vi "ATReadErds.vi"(0 "GEA2 Reference In":refnum<k24>, 5 "Destination":string, 7 "Erd Number":string, 11 "Error In":errorcluster) -> (4 "GEA2 Reference Out":refnum<k24>, 8 "ERD Data Out":string, 15 "Error Out":errorcluster)   [LabVIEW 2021]
uses:
  D:/Common/LabVIEW GEA2 Toolkit/source/GEA3 DLL Source/GeaCommunication.dll
  Common/LabVIEW GEA2 Toolkit/source/GEA3 DLL Source/GeaCommunication.dll
  Common/LabVIEW GEA2 Toolkit/GEA3/type defs/Data Type.ctl
  Common/LabVIEW GEA2 Toolkit/GEA3/library/GEA2_Toolkit.lvlib
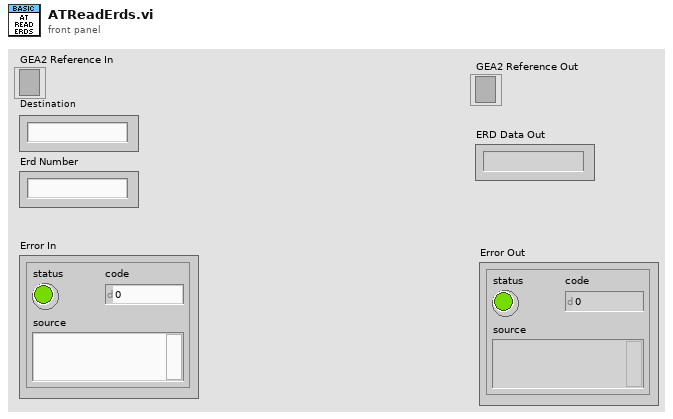
[diagram p1: front panel]
types:
  T1 = typedef "Data Type.ctl" = enum16{"string", "boolean", "uint8_t", "uint16_t", "uint32_t", "uint64_t", "int8_t", "int16_t", "int32_t", "int64_t"}
  T2 = cluster{"ERD Data Out[0]":cluster{"ERD Number":u16, "Data":string}, "ERD Data Out[1]":cluster{"ERD Number":u16, "Data":string}, "ERD Data Out[2]":cluster{"ERD Number":u16, "Data":string}, "ERD Data Out[3]":cluster{"ERD Number":u16, "Data":string}, "ERD Data Out[4]":cluster{"ERD Number":u16, "Data":string}, "ERD Data Out[5]":cluster{"ERD Number":u16, "Data":string}, "ERD Data Out[6]":cluster{"ERD Number":u16, "Data":string}, "ERD Data Out[7]":cluster{"ERD Number":u16, "Data":string}, "ERD Data Out[8]":cluster{"ERD Number":u16, "Data":string}}
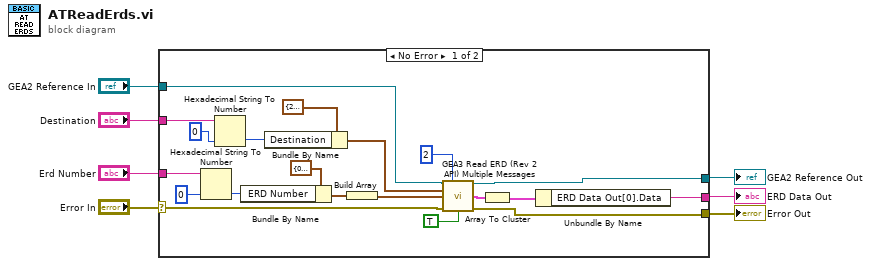
[diagram p0: block diagram]
diagram:
  n1 = case shown="No Error" "Error In" {
    selector: "Error In" -> [w12 w29]
    tunnel: "GEA2 Reference In" -> [w16 w28]
    tunnel: "Destination" -> [w20 _]
    tunnel: "Erd Number" -> [w19 _]
    tunnel: [w15 w28] -> w4
    tunnel: [w17 _] -> w3
    tunnel: [w13 w29] -> w1
    frame No Error {
      n2 = Hexadecimal String To Number(string=w19, default (0uL)=u16 0 ("ERD Number")) -> (number=w23:u16)  [unwired: 1 in, 1 out]
      n3 = Hexadecimal String To Number(string=w20, default (0uL)=u8 0 ("Destination")) -> (number=w26:u8)  [unwired: 1 in, 1 out]
      n4 = Bundle By Name(cluster=cluster{"ERD Number":u16, "Data Type":T1} {"ERD Number"=0, "Data Type"=enum."string"} ("ERD Read Data In"), "ERD Number"=w23) -> (w21:cluster{"ERD Number":u16, "Data Type":T1})
      n5 = Bundle By Name(cluster=cluster{"Source":u8, "Destination":u8} {"Source"=229, "Destination"=0} ("GEA Inputs"), "Destination"=w26) -> (w10:cluster{"Source":u8, "Destination":u8})
      n6 = Build Array(w21) -> (w11:cluster{"ERD Number":u16, "Data Type":T1}[])
      n7 = call "GEA3 Read ERD (Rev 2 API) Multiple Messages.vi"("GEA2 Reference In"=w16, "Retry Count"=2, "GEA Inputs"=w10, "Read ERD List"=w11, "Error In"=w12, "Verify ERD Response?"=TRUE) -> ("GEA2 Reference Out"=w15:refnum<k24>, "ERD Data Out"=w14:cluster{"ERD Number":u16, "Data":string}[], "Error Out"=w13:errorcluster)  [unwired: 6 in, 1 out]
      n8 = Array To Cluster(array=w14) -> (cluster=w18:T2)
      n9 = Unbundle By Name(w18) -> ("ERD Data Out[0].Data"=w17:string)
    }
    frame Error {
    }
  }
  "GEA2 Reference Out" <- w4
  "ERD Data Out" <- w3
  "Error Out" <- w1
